vi "Main.vi"(11 "Module Admin":refnum<class "Delacor_lib_QMH_Cloneable Module Admin.lvclass">) -> ()   [LabVIEW 2020, in "Mensajes.lvlib"]
doc: "This template is based off of the Queued Message Handler design pattern and the Queued Message Handler project template that ships with LabVIEW.\n\nThe main difference is that the queue is private to this module and communication between modules is performed via Broadcast and Request events.\n\nRequest events are wrapped in public API methods and are handled in the Event Handling Loop (EHL) of this VI. Any module can register for Broadcast events sent by this module. The EHL generates messages based on user interface actions.\n\nThe Message Handling Loop (MHL) processes messages generated by the EHL, or by other messages. The messages are string values, so new messages can be added easily to the Message Cases case structure in the MHL. Each message cluster can also provide an optional value for Message Data, which is a variant that can be converted to whatever message-specific data is required.\n_____\nBased on DQMH Dev Tools: Project Template 7.1.0.1503."
uses:
  Mensajes.lvlib
  <vilib>/Delacor/Delacor QMH/Libraries/Cloneable Module Admin_class/Delacor_lib_QMH_Cloneable Module Admin.lvclass
  C:/Program Files (x86)/National Instruments/LabVIEW 2024/vi.lib/Delacor/Delacor QMH/Libraries/Module Admin_class/Delacor_lib_QMH_Module Admin.lvclass
  Module Data--cluster.ctl
  <vilib>/Delacor/Delacor QMH/Libraries/Cloneable Module Admin_class/Delacor_lib_QMH_Cloneable Module Admin.lvclass/Delacor_lib_QMH_Cloneable Module Admin.ctl
  Stop Argument--cluster.ctl
  <vilib>/Delacor/Delacor QMH/Libraries/Message Queue_class/Delacor_lib_QMH_Message Queue.lvclass/Delacor_lib_QMH_Message Queue.ctl
  <vilib>/Delacor/Delacor QMH/Libraries/Module Admin_class/Delacor_lib_QMH_Module Admin.lvclass/Delacor_lib_QMH_Module Admin.ctl
  Draw FP in Subpanel Argument--cluster.ctl
  Remove From Subpanel Argument--cluster.ctl
  Set Font Settings Argument--cluster.ctl
  <vilib>/Utility/miscctls.llb/LVFontTypeDef.ctl
  Set Message Argument--cluster.ctl
  Append String Argument--cluster.ctl
  DisplayStyle--enum.ctl
  Set Display Style Argument--cluster.ctl
  <vilib>/Utility/miscctls.llb/LVPointTypeDef.ctl
  <vilib>/Delacor/Delacor QMH/Libraries/Cloneable Module Admin_class/Delacor_lib_QMH_Get Module ID.vi
  <vilib>/Delacor/Delacor QMH/Libraries/Message Queue_class/Delacor_lib_QMH_Enqueue Message (Single).vi
  <vilib>/Delacor/Delacor QMH/Libraries/Module Admin_class/Delacor_lib_QMH_Get External Launch.vi
  <vilib>/Delacor/Delacor QMH/Libraries/Message Queue_class/Delacor_lib_QMH_Message Queue.lvclass
panel:
  out "Message":string
  out "error out":errorcluster
  out "Status":string
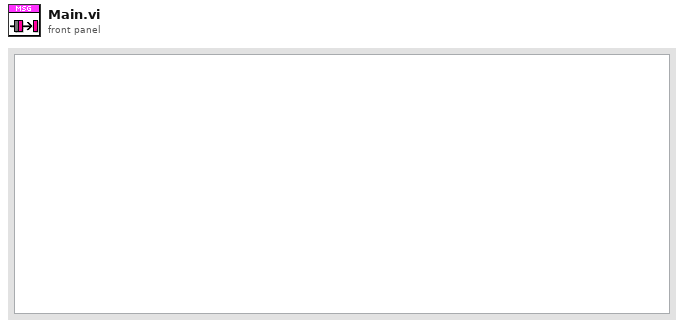
[diagram p1: front panel]
types:
  T1 = typedef "Mensajes.lvlib/Request Events--cluster.ctl" = cluster{"Stop Module":refnum<user-event>, "Show Panel":refnum<user-event>, "Hide Panel":refnum<user-event>, "Show Diagram":refnum<user-event>, "Get Module Execution Status":refnum<user-event>, "Draw FP in Subpanel":refnum<user-event>, "Remove From Subpanel":refnum<user-event>, "Set Font Settings":refnum<user-event>, "Set Message":refnum<user-event>, "Append String":refnum<user-event>, "Set Display Style":refnum<user-event>}
  T2 = typedef "Mensajes.lvlib/Module Data--cluster.ctl" = cluster{"Status":string, "Sub Panel":refnum<vi>, "Message Ref":refnum<vi>}
  T3 = enum32{"invalid lock state", "Not Locked", "Locked (No Password)", "Password-protected"}
  T4 = typedef "Mensajes.lvlib/Stop Argument--cluster.ctl" = cluster{"Module ID":i32, "Origin":string, "Exit via Stop Module Req?":bool, "Wait for Module to stop?":bool}
  T5 = typedef "Mensajes.lvlib/Draw FP in Subpanel Argument--cluster.ctl" = cluster{"Module ID":i32, "Sub Panel":refnum<vi>}
  T6 = typedef "Mensajes.lvlib/Remove From Subpanel Argument--cluster.ctl" = cluster{"Module ID":i32, "Boolean":bool}
  T7 = typedef "Mensajes.lvlib/Set Font Settings Argument--cluster.ctl" = cluster{"Module ID":i32, "Text.Font":T8}
  T8 = typedef "LVFontTypeDef.ctl" = cluster{"Font Name":string, "Size":u16, "Bold":bool, "Italic":bool, "Underline":bool, "Strikeout":bool, "Color":u32}
  T9 = typedef "Mensajes.lvlib/Set Message Argument--cluster.ctl" = cluster{"Module ID":i32, "Message":string}
  T10 = typedef "Mensajes.lvlib/Append String Argument--cluster.ctl" = cluster{"Module ID":i32, "String to Append":string}
  T11 = typedef "Mensajes.lvlib/DisplayStyle--enum.ctl" = enum16{"Normal", "Backslash", "Password", "Hexadecimal"}
  T12 = typedef "Mensajes.lvlib/Set Display Style Argument--cluster.ctl" = cluster{"Module ID":i32, "Display Style":T11}
  T13 = typedef "LVPointTypeDef.ctl" = cluster{"Horizontal":i16, "Vertical":i16}
  T14 = enum32{"Invalid", "Standard", "Closed", "Hidden", "Minimized", "Maximized"}
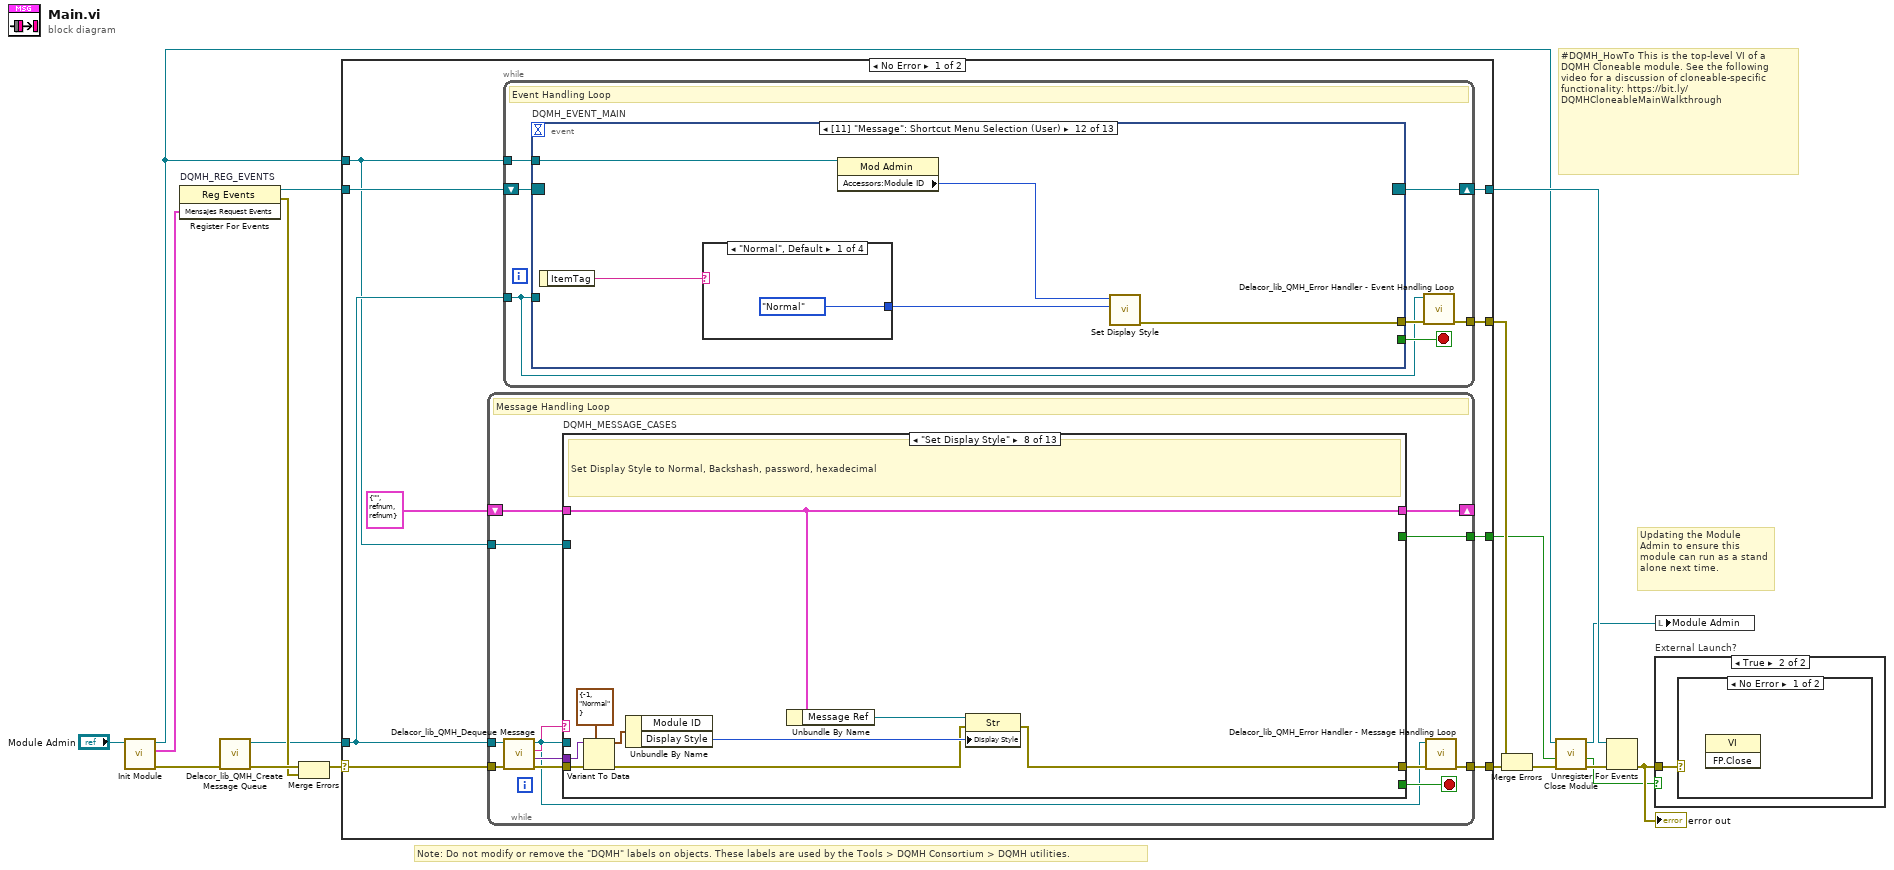
[diagram p0: block diagram]
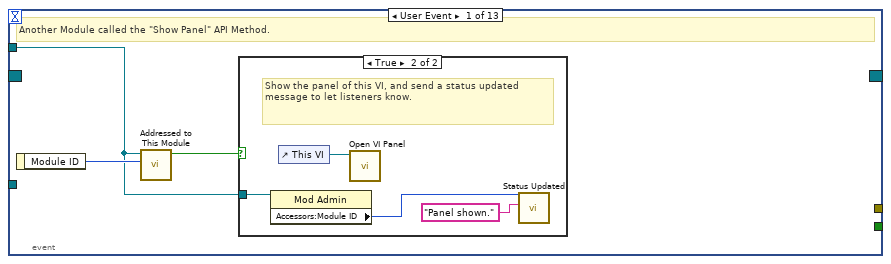
[diagram p2: hidden frame]
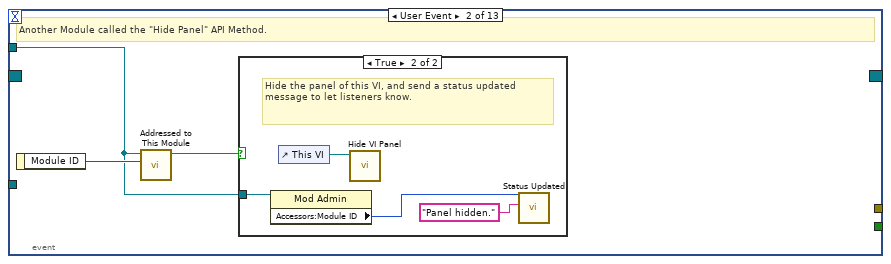
[diagram p4: hidden frame]
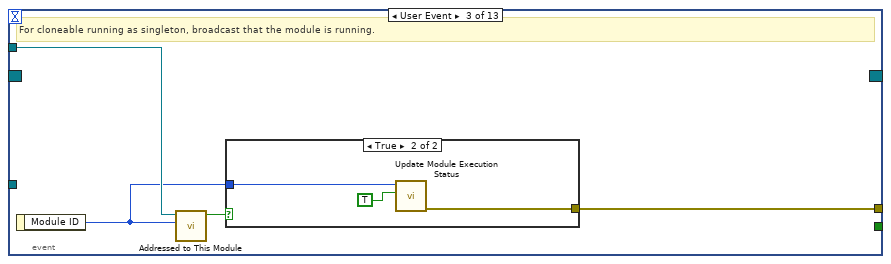
[diagram p6: hidden frame]
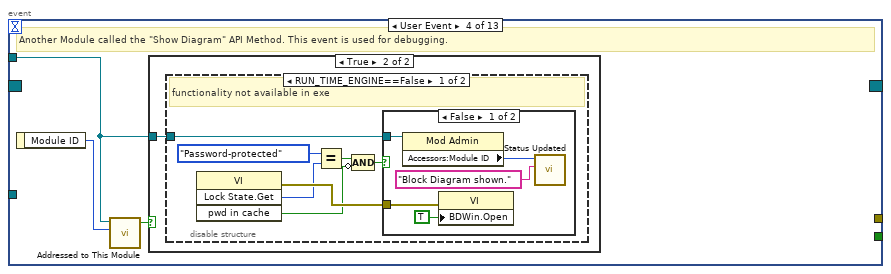
[diagram p8: hidden frame]
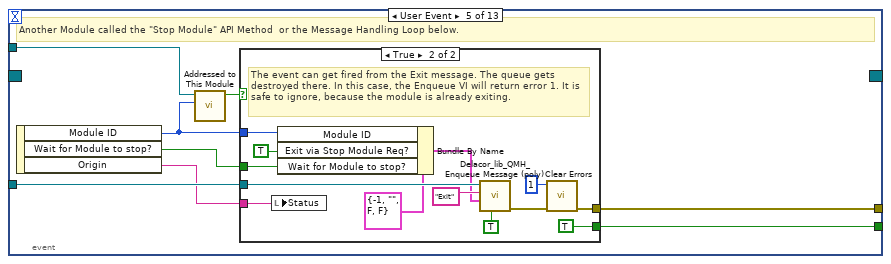
[diagram p12: hidden frame]
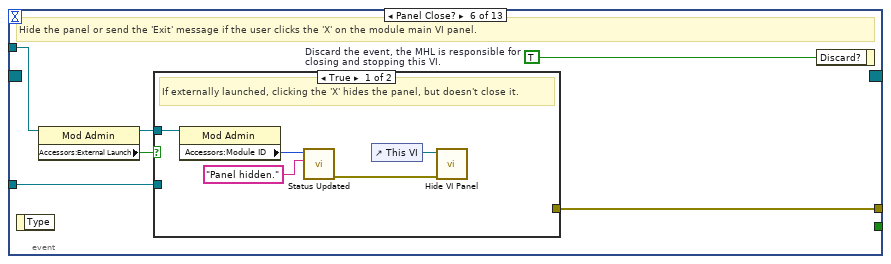
[diagram p14: hidden frame]
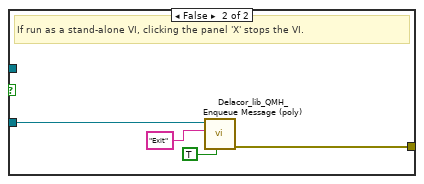
[diagram p15: hidden frame]
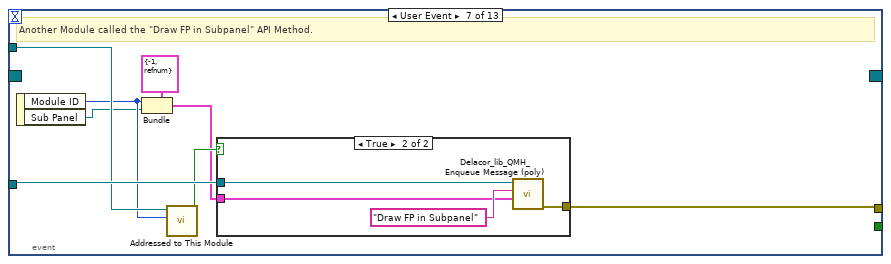
[diagram p16: hidden frame]
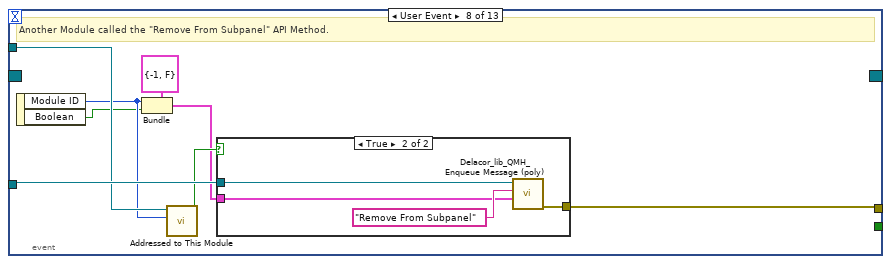
[diagram p18: hidden frame]
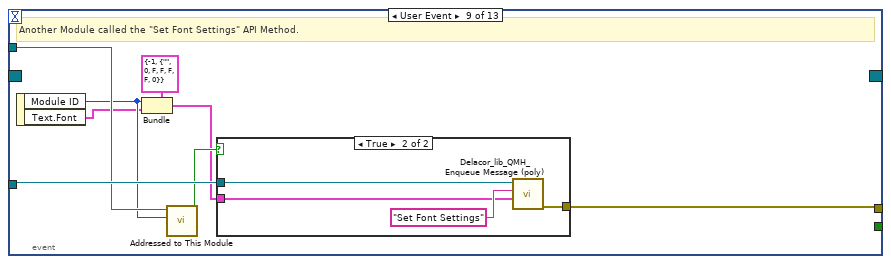
[diagram p20: hidden frame]
diagram:
  # "#DQMH_HowTo This is the top-level VI of a DQMH Cloneable module. See the following video for a discussion of cloneable-specific functionality: https://bit.ly/DQMHCloneableMainWalkthrough"
  # "Note: Do not modify or remove the \"DQMH\" labels on objects. These labels are used by the Tools > DQMH Consortium > DQMH utilities."
  # "Updating the Module Admin to ensure this module can run as a stand alone next time."
  n1 = call "Init Module.vi"("Cloneable Module Admin in"="Module Admin") -> ("error out"=w15:errorcluster, "Mensajes Request Events"=w7:T1, "Cloneable Module Admin out"=w4:refnum<class "Delacor_lib_QMH_Cloneable Module Admin.lvclass">)  [unwired: 8 in]
  n2 = register-events "DQMH_REG_EVENTS"(w7) -> (reference out=w8:refnum<event-registration>, error out=w10:errorcluster)  [unwired: 2 in]
  n3 = call <vilib>:"Delacor_lib_QMH_Create Message Queue.vi"("error in"=w15) -> ("error out"=w12:errorcluster, "Message Queue"=w6:refnum<class "Delacor_lib_QMH_Message Queue.lvclass">)  [unwired: 9 in]
  n4 = Merge Errors(w12, w10) -> (w11:errorcluster)
  n5 = case shown="No Error" w11 {
    selector: w11 -> [w25 w375]
    tunnel: [w27 w374] -> w16
    tunnel: [w24 w373] -> w9
    tunnel: w8 -> [w22 w373]
    tunnel: w6 -> [w21 w366]
    tunnel: [w26 _] -> w17
    tunnel: w4 -> [w20 w369]
    tunnel: [w19 _] -> w2
    frame No Error {
      n6 = while {
        tunnel: w21 -> [w189]
        shift-right: [w196] -> _
        shift-left: T2 {"Status"="", "Sub Panel"=refnum, "Message Ref"=refnum} ("Data Cluster") -> [w197]
        tunnel: w25 -> [w200]
        tunnel: [w198] -> w27
        tunnel: w20 -> [w191]
        tunnel: [w190] -> w19
        stop <- w195 stop-if-true
        # "Message Handling Loop"
        n7 = call-dynamic "Delacor_lib_QMH_Dequeue Message.vi"("error in"=w200, "Message Queue in"=w189) -> ("error out"=w199:errorcluster, "Message Data"=w193:variant, "Message"=w194:string, "Message Queue out"=w192:refnum<class "Delacor_lib_QMH_Message Queue.lvclass">)  [unwired: 6 in]
        n8 = case "DQMH_MESSAGE_CASES" shown="\"Set Display Style\"" w194 {
          selector: w194 -> [_ _ _ _ _ _ _ _ _ _ _ _ w355]
          tunnel: w192 -> [_ _ _ _ _ _ _ _ _ _ w319 w347 _]
          tunnel: w199 -> [w221 w225 w244 w264 w279 w290 w303 w312 w315 w317 w329 w353 w364]
          tunnel: [w219 w225 w240 w262 w274 w288 w298 w306 w314 w317 w325 w348 w365] -> w201
          tunnel: w197 -> [w212 w224 w230 w256 w272 w289 w297 w305 w313 w316 w323 w337 w362]
          tunnel: [w211 w224 w231 w252 w272 w289 w297 w305 w313 w316 w323 w337 w362] -> w196
          tunnel: [_ _ _ _ _ _ _ _ _ _ _ w346 _] -> w195
          tunnel: w193 -> [_ _ w239 w261 w278 w287 w302 w311 _ _ w322 w344 _]
          tunnel: w191 -> [w207 _ w228 w255 _ w284 w294 _ _ _ w321 w339 w361]
          tunnel: [_ _ _ _ _ _ _ _ _ _ _ w342 _] -> w190
          frame "Initialize" {
            w204 = "Initial Message" ("Initial Message")
            # "Initialize - Any operation that needs to be done before the module can receive messages. Synchronize Caller Events.vi will inform Start Module.vi that the module has launched and is ready to receive messages. Module Did Init.vi will broadcast that the module initialized."
            n9 = call "Synchronize Caller Events.vi"("error in"=w221, "Module Admin"=w207) -> ("error out"=w220:errorcluster, "Module Admin out"=w206:refnum<class "Delacor_lib_QMH_Cloneable Module Admin.lvclass">)  [unwired: 8 in]
            n10 = property on="Property Node" class="Mod Admin"(reference=w206) -> ("Accessors:Module ID"=w203:i32, "Accessors:External Launch"=w208:bool)  [unwired: 1 in, 2 out]
            n11 = call "Module Name--constant.vi"("Module ID"=w203) -> ("Module Name"=w216:string)  [unwired: 10 in]
            n12 = property on="Property Node" class="VI"("Front Panel.Title"=w216) -> (reference out=w218:refnum<vi>, error out=w223:errorcluster)  [unwired: 2 in]
            n13 = Select(t=T14."Hidden" ("State"), s=w208, f=T14."Standard" ("State")) -> (s? t:f=w213:T14)
            n14 = control-ref of="Message"() -> (w202:refnum<vi>)
            n15 = invoke on="Invoke Node" class="VI" method="FP.Open"(reference=w218, error in=w223, "State"=w213) -> (reference out=w217:refnum<vi>, error out=w222:errorcluster)  [unwired: 2 in, 3 out]
            n16 = Bundle By Name(cluster=w212, "Message Ref"=w202, "Status"=w204) -> (w211:T2)
            n17 = invoke on="Invoke Node" class="VI" method="FP.Center"(reference=w217, error in=w222) -> ()  [unwired: 1 in, 3 out]
            n18 = property on="Pane" class="Pane"("Origin"=T13 {"Horizontal"=0, "Vertical"=0}) -> ()  [unwired: 2 in, 2 out]
            n19 = call "Module Name--constant.vi"("Module ID"=w203) -> ("Module Name"=w209:string)  [unwired: 10 in]
            n20 = call "Module Did Init.vi"("error in"=w220, "Initialized?"=TRUE, "Origin"=w209, "Module ID"=w203) -> ("error out"=w219:errorcluster)  [unwired: 7 in]
            "Status" <- w204
          }
          frame "---Module Specific---" {
            # "Separator -- The following cases handle messages specific to this Module."
          }
          frame "Draw FP in Subpanel" {
            # "Draw FP in Subpanel"
            n21 = Variant To Data(error in=w244, type=T5 {"Module ID"=-1, "Sub Panel"=refnum} ("Draw FP in Subpanel Argument"), Variant=w239) -> (data=w237:T5, error out=w241:errorcluster)
            n22 = property class="Mod Admin"(reference=w228) -> ("Accessors:Module ID"=w227:i32)  [unwired: 1 in, 2 out]
            n23 = Unbundle By Name(w237) -> ("Sub Panel"=w229:refnum<vi>)
            n24 = control-ref of="This VI"() -> (w234:refnum<vi>)
            n25 = property class="VI"(reference=w234, error in=w241) -> (reference out=w233:refnum<vi>, error out=w242:errorcluster, "FP.State"=w232:T14)
            n26 = case shown="\"Closed\"" w232 {
              tunnel: [w245 w248] -> w235
              tunnel: [w246 w250] -> w243
              tunnel: w242 -> [w246 w249]
              tunnel: w233 -> [w245 w247]
              frame "Closed" {
              }
              frame "Standard", Default {
                n27 = invoke class="VI" method="FP.Close"(reference=w247, error in=w249) -> (reference out=w248:refnum<vi>, error out=w250:errorcluster)  [unwired: 1 in, 1 out]
              }
            }
            n28 = invoke class="SubPnl" method="Insert VI"(reference=w229, error in=w243, "VI Ref"=w235) -> (reference out=w236:refnum<vi>, error out=w240:errorcluster)  [unwired: 1 in, 2 out]
            n29 = call "Status Updated.vi"("error in"=w240, "Status"="Front Panel Inserted in Subpanel", "Module ID"=w227) -> ()  [unwired: 8 in, 1 out]
            n30 = Bundle By Name(cluster=w230, "Sub Panel"=w236) -> (w231:T2)
          }
          frame "Remove From Subpanel" {
            # "Remove From Subpanel"
            n31 = Variant To Data(error in=w264, type=T6 {"Module ID"=-1, "Boolean"=FALSE} ("Remove From Subpanel Argument"), Variant=w261) -> (data=w259:T6, error out=w263:errorcluster)
            n32 = Unbundle By Name(w259) -> ()  [unwired: 2 out]
            n33 = property class="Mod Admin"(reference=w255) -> ("Accessors:Module ID"=w254:i32)  [unwired: 1 in, 2 out]
            n34 = Unbundle By Name(w256) -> ("Sub Panel"=w258:refnum<vi>)
            n35 = Not A Number/Path/Refnum?(number/path/refnum=w258) -> (NaN/Path/Refnum?=w257:bool)
            n36 = case shown="False" w257 {
              tunnel: w263 -> [w268 w270]
              tunnel: [w267 w270] -> w262
              tunnel: w258 -> [w266 _]
              tunnel: ["Panel Removed from Subpanel" "This module has not been inserted into the subpanel"] -> w253
              frame False {
                n37 = invoke class="SubPnl" method="Remove VI"(reference=w266, error in=w268) -> (error out=w267:errorcluster)  [unwired: 1 in, 2 out]
              }
              frame True {
              }
            }
            n38 = Bundle By Name(cluster=w256, "Sub Panel"=refnum<vi> refnum) -> (w252:T2)
            n39 = call "Status Updated.vi"("error in"=w262, "Status"=w253, "Module ID"=w254) -> ()  [unwired: 8 in, 1 out]
          }
          frame "Set Font Settings" {
            # "Set Font Name, Size, Bold, Italic, Underline, Strikeout, and Color"
            n40 = Variant To Data(error in=w279, type=T7 {"Module ID"=-1, "Text.Font"={"Font Name"="", "Size"=0, "Bold"=FALSE, "Italic"=FALSE, "Underline"=FALSE, "Strikeout"=FALSE, "Color"=0}} ("Set Font Settings Argument"), Variant=w278) -> (data=w276:T7, error out=w275:errorcluster)
            n41 = Unbundle By Name(w276) -> ("Text.Font"=w273:T8)  [unwired: 1 out]
            n42 = Unbundle By Name(w272) -> ("Message Ref"=w271:refnum<vi>)
            n43 = property class="Str"(reference=w271, error in=w275, "Text.Font"=w273) -> (error out=w274:errorcluster)  [unwired: 1 out]
          }
          frame "Set Message" {
            # "Set Message"
            n44 = Variant To Data(error in=w290, type=T9 {"Module ID"=-1, "Message"=""} ("Set Message Argument"), Variant=w287) -> (data=w285:T9, error out=w288:errorcluster)
            n45 = property class="Mod Admin"(reference=w284) -> ("Accessors:Module ID"=w283:i32)  [unwired: 1 in, 2 out]
            n46 = Unbundle By Name(w285) -> ("Message"=w282:string)
            "Message" <- w282
            n47 = Format Into String(format string="Message Set: %s", w282) -> (resulting string=w281:string)  [unwired: 2 in, 1 out]
            n48 = call "Status Updated.vi"("Status"=w281, "Module ID"=w283) -> ()  [unwired: 9 in, 1 out]
          }
          frame "Append String" {
            # "Append String"
            n49 = Variant To Data(error in=w303, type=T10 {"Module ID"=-1, "String to Append"=""} ("Append String Argument"), Variant=w302) -> (data=w300:T10, error out=w299:errorcluster)
            n50 = Unbundle By Name(w300) -> ("String to Append"=w293:string)  [unwired: 1 out]
            n51 = property class="Mod Admin"(reference=w294) -> ("Accessors:Module ID"=w295:i32)  [unwired: 1 in, 2 out]
            n52 = Unbundle By Name(w297) -> ("Message Ref"=w296:refnum<vi>)
            n53 = Format Into String(format string="Appending String: %s", w293) -> (resulting string=w292:string)  [unwired: 2 in, 1 out]
            n54 = invoke class="Str" method="Append String"(reference=w296, error in=w299, "string"=w293) -> (error out=w298:errorcluster)  [unwired: 1 in, 3 out]
            n55 = call "Status Updated.vi"("Status"=w292, "Module ID"=w295) -> ()  [unwired: 9 in, 1 out]
          }
          frame "Set Display Style" {
            # "Set Display Style to Normal, Backshash, password, hexadecimal"
            n56 = Variant To Data(error in=w312, type=T12 {"Module ID"=-1, "Display Style"=enum."Normal"} ("Set Display Style Argument"), Variant=w311) -> (data=w309:T12, error out=w307:errorcluster)
            n57 = Unbundle By Name(w309) -> ("Display Style"=w308:T11)  [unwired: 1 out]
            n58 = Unbundle By Name(w305) -> ("Message Ref"=w304:refnum<vi>)
            n59 = property class="Str"(reference=w304, error in=w307, "Display Style"=w308) -> (error out=w306:errorcluster)  [unwired: 1 out]
          }
          frame "---Copy This Frame---" {
            # "Duplicate this frame when creating new messages.  Change this comment in the duplicated frame to describe this message."
            n60 = Merge Errors(w315) -> (w314:errorcluster)
          }
          frame "---Exit and Error Handling---" {
            # "Separator - the following cases handle errors and exit messages."
          }
          frame "Error" {
            # "#DQMH_CodeRecommended - If the module is running in standalone mode (External Launch = FALSE), this code will pop up an error dialog and call the 'Exit' message if an error occurs. Add more fine-grained error management here."
            # "Error - Check the error message data and respond accordingly. This message is sent by the \"Error Handler\" VIs at the end of each loop in this application."
            n61 = property on="Property Node" class="Mod Admin"(reference=w321) -> ("Accessors:External Launch"=w320:bool, "Accessors:Module ID"=w318:i32)  [unwired: 1 in, 2 out]
            n62 = Variant To Data(error in=w329, type=errorcluster {"status"=FALSE, "code"=0, "source"=""} ("error constant"), Variant=w322) -> (data=w324:errorcluster, error out=w327:errorcluster)
            n63 = local write "error out"(w324) -> ()
            n64 = call "Error Reported.vi"("Error"=w324, "Module ID"=w318) -> ()  [unwired: 9 in, 1 out]
            n65 = case shown="False" w320 {
              tunnel: [w334 _] -> w326
              tunnel: w319 -> [w332 _]
              tunnel: w324 -> [w333 _]
              frame False {
                n66 = disable-structure shown="Default" {
                  disable-tunnel: w333 -> [w335 _]
                  frame condition #0 (active) {
                    # "If the module is running standalone, then pop up an error dialog and call the \"Exit\" message."
                    n67 = call <vilib>:"Simple Error Handler.vi"("error in (no error)"=w335) -> ()  [unwired: 4 in, 5 out]
                  }
                  frame condition #1 {
                    # "To prevent the Simple Error Handler VI from being loaded (e.g. when deploying to a Real-Time target), add the Conditional Disable Symbol \"DQMH_Disable_SEH\" to your project and set it to TRUE."
                  }
                }
                n68 = call-poly <vilib>:"Delacor_lib_QMH_Enqueue Message (poly).vi"("Priority Message? (F)"=TRUE, "Message"="Exit", "Message Queue in"=w332) -> ("error out"=w334:errorcluster)  [unwired: 7 in, 1 out]
              }
              frame True {
                # "If the module was launched externally, calling the Error Reported broadcast VI is the only action performed by the \"Error\" message. The module's caller can then process the error appropriately."
              }
            }
            n69 = Merge Errors(w327, w326) -> (w325:errorcluster)
          }
          frame "Exit" {
            w345 = 91  # 91: not all Exit messages will have an argument
            w346 = TRUE  # Stop the VI
            # "Release the message queue reference"
            # "#DQMH_CodeNeeded - Add any required cleanup code here."
            # "Exit - Exit the application."
            n70 = Variant To Data(error in=w353, type=T4 {"Module ID"=-1, "Origin"="", "Exit via Stop Module Req?"=FALSE, "Wait for Module to stop?"=FALSE} ("Stop Argument"), Variant=w344) -> (data=w341:T4, error out=w349:errorcluster)
            n71 = call <vilib>:"Clear Errors.vi"("error in (no error)"=w349, "specific error code to clear (0: all)"=w345) -> ("error out"=w352:errorcluster)  [unwired: 4 in, 1 out]
            n72 = property on="Property Node" class="Mod Admin"(reference=w339) -> ("Accessors:Module ID"=w338:i32)  [unwired: 1 in, 2 out]
            n73 = control-ref of="This VI"() -> (w340:refnum<vi>)
            n74 = call-dynamic "Delacor_lib_QMH_Release Message Queue.vi"("error in"=w352, "Message Queue"=w347) -> ("error out"=w351:errorcluster)  [unwired: 9 in]
            n75 = call "Handle Exit.vi"("Stop Argument"=w341, "Module Admin in"=w339, "VI reference"=w340) -> ("error out"=w350:errorcluster, "Wait for Stop?"=w342:bool)  [unwired: 7 in]
            n76 = Merge Errors(w351, w350) -> (w348:errorcluster)
            n77 = Unbundle By Name(w337) -> ("Sub Panel"=w336:refnum<vi>)
            n78 = call "Error Reported.vi"("Error"=w348, "Module ID"=w338) -> ()  [unwired: 9 in, 1 out]
            n79 = invoke class="SubPnl" method="Remove VI"(reference=w336) -> ()  [unwired: 2 in, 3 out]
          }
          frame Default {
            # "'Default' case only runs if there is a message that isn't defined in any of the other cases.  Output a programming error."
            n80 = property on="Property Node" class="Mod Admin"(reference=w361) -> ("Accessors:Module ID"=w360:i32)  [unwired: 1 in, 2 out]
            n81 = call "Module Name--constant.vi"("Module ID"=w360) -> ("Module Name"=w354:string)  [unwired: 10 in]
            n82 = Format Into String(format string="The invalid message string \"%s\" was received in the Message Handling Loop for module \"%s\".", w355, w354) -> (resulting string=w357:string)  [unwired: 2 in, 1 out]
            n83 = call <vilib>:"Error Cluster From Error Code.vi"("show call chain? (False)"=TRUE, "error message (\"\")"=w357, "error code (0)"=1) -> ("error out"=w363:errorcluster)  [unwired: 6 in]
            n84 = Merge Errors(w364, w363) -> (w365:errorcluster)
          }
        }
        n85 = call-dynamic "Delacor_lib_QMH_Error Handler - Message Handling Loop.vi"("error in"=w201, "Message Queue in"=w192) -> ("dup error in"=w198:errorcluster)  [unwired: 8 in, 1 out]
      }
      n86 = while {
        tunnel: w21 -> [w28]
        shift-right: [w31] -> w24
        shift-left: w22 -> [w32]
        tunnel: [w33] -> w26
        tunnel: w20 -> [w29]
        stop <- w30 stop-if-true
        # "Event Handling Loop"
        n87 = event "DQMH_EVENT_MAIN" shown="[11] \"Message\": Shortcut Menu Selection (User)" {
          selector: w32 -> [_ _ _ _ _ _ _ _ _ _ _ _ _]
          dyn-events: [_ _ _ _ _ _ _ _ _ _ _ _ _] -> w31
          timeout: _ -> [_ _ _ _ _ _ _ _ _ _ _ _ _]
          tunnel: [_ _ _ _ w75 _ _ _ _ _ _ _ _] -> w30
          tunnel: w28 -> [_ _ _ _ w78 w95 w114 w126 w139 w151 w163 _ w184]
          tunnel: [_ _ w52 _ w79 w98 w115 w127 w132 w144 w156 w168 w177] -> w34
          tunnel: w29 -> [w35 w42 w50 w56 w77 w96 w112 w124 w137 w149 w161 w172 w182]
          event User Event {
            # "Another Module called the \"Show Panel\" API Method."
            n88 = event-data() -> ("Module ID"=w36:i32)  [unwired: 1 in]
            n89 = call "Addressed to This Module.vi"("Module ID from Argument"=w36, "Module Admin"=w35) -> ("Addressed to this instance?"=w37:bool)  [unwired: 8 in, 1 out]
            n90 = case shown="True" w37 {
              tunnel: w35 -> [_ w39]
              frame False {
              }
              frame True {
                # "Show the panel of this VI, and send a status updated message to let listeners know."
                n91 = property on="Property Node" class="Mod Admin"(reference=w39) -> ("Accessors:Module ID"=w38:i32)  [unwired: 1 in, 2 out]
                n92 = control-ref of="This VI"() -> (w41:refnum<vi>)
                n93 = call "Open VI Panel.vi"("VI"=w41) -> ()  [unwired: 10 in, 1 out]
                n94 = call "Status Updated.vi"("Status"="Panel shown." ("format string"), "Module ID"=w38) -> ()  [unwired: 9 in, 1 out]
              }
            }
          }
          event User Event {
            # "Another Module called the \"Hide Panel\" API Method."
            n95 = event-data() -> ("Module ID"=w43:i32)  [unwired: 1 in]
            n96 = call "Addressed to This Module.vi"("Module ID from Argument"=w43, "Module Admin"=w42) -> ("Addressed to this instance?"=w44:bool)  [unwired: 8 in, 1 out]
            n97 = case shown="True" w44 {
              tunnel: w42 -> [_ w46]
              frame False {
              }
              frame True {
                # "Hide the panel of this VI, and send a status updated message to let listeners know."
                n98 = property on="Property Node" class="Mod Admin"(reference=w46) -> ("Accessors:Module ID"=w45:i32)  [unwired: 1 in, 2 out]
                n99 = control-ref of="This VI"() -> (w48:refnum<vi>)
                n100 = call "Hide VI Panel.vi"("VI"=w48) -> ()  [unwired: 10 in, 1 out]
                n101 = call "Status Updated.vi"("Status"="Panel hidden." ("format string"), "Module ID"=w45) -> ()  [unwired: 9 in, 1 out]
              }
            }
          }
          event User Event {
            # "For cloneable running as singleton, broadcast that the module is running."
            n102 = event-data() -> ("Module ID"=w49:i32)  [unwired: 1 in]
            n103 = call "Addressed to This Module.vi"("Module ID from Argument"=w49, "Module Admin"=w50) -> ("Addressed to this instance?"=w51:bool)  [unwired: 8 in, 1 out]
            n104 = case shown="True" w51 {
              tunnel: [_ w55] -> w52
              tunnel: w49 -> [_ w54]
              frame False {
              }
              frame True {
                n105 = call "Update Module Execution Status.vi"("Running?"=TRUE, "Module ID"=w54) -> ("error out"=w55:errorcluster)  [unwired: 9 in]
              }
            }
          }
          event User Event {
            # "Another Module called the \"Show Diagram\" API Method. This event is used for debugging."
            n106 = event-data() -> ("Module ID"=w57:i32)  [unwired: 1 in]
            n107 = call "Addressed to This Module.vi"("Module ID from Argument"=w57, "Module Admin"=w56) -> ("Addressed to this instance?"=w58:bool)  [unwired: 8 in, 1 out]
            n108 = case shown="True" w58 {
              tunnel: w56 -> [_ w59]
              frame False {
              }
              frame True {
                n109 = disable-structure shown="RUN_TIME_ENGINE==False" {
                  disable-tunnel: w59 -> [w60 _]
                  frame condition #0 (active) {
                    # "functionality not available in exe"
                    n110 = invoke on="Invoke Node" class="VI" method="Lock State.Get"() -> (error out=w66:errorcluster, "Get Lock State"=w65:T3, "pwd in cache"=w62:bool)  [unwired: 4 in, 1 out]
                    n111 = Equal?(x=T3."Password-protected", y=w65) -> (x = y?=w63:bool)
                    n112 = Compound Arithmetic op=AND(w63, invert w62) -> (w61:bool)
                    n113 = case shown="False" w61 {
                      tunnel: w66 -> [w71 _]
                      tunnel: w60 -> [w68 _]
                      frame False {
                        n114 = property on="Property Node" class="Mod Admin"(reference=w68) -> ("Accessors:Module ID"=w67:i32)  [unwired: 1 in, 2 out]
                        n115 = property on="Property Node" class="VI"(error in=w71, "BDWin.Open"=TRUE ("Block Diagram Window:Open")) -> ()  [unwired: 1 in, 2 out]
                        n116 = call "Status Updated.vi"("Status"="Block Diagram shown." ("format string"), "Module ID"=w67) -> ()  [unwired: 9 in, 1 out]
                      }
                      frame True {
                        # "Password-protected VI, and the password is not in the cache. Do not show the diagram."
                      }
                    }
                  }
                  frame condition #1 {
                  }
                }
              }
            }
          }
          event User Event {
            # "Another Module called the \"Stop Module\" API Method  or the Message Handling Loop below."
            n117 = event-data() -> ("Module ID"=w73:i32, "Wait for Module to stop?"=w74:bool, "Origin"=w72:string)  [unwired: 1 in]
            n118 = call "Addressed to This Module.vi"("Module ID from Argument"=w73, "Module Admin"=w77) -> ("Addressed to this instance?"=w76:bool)  [unwired: 8 in, 1 out]
            n119 = case shown="True" w76 {
              tunnel: [_ w91] -> w79
              tunnel: w78 -> [_ w87]
              tunnel: [_ TRUE] -> w75
              tunnel: w74 -> [_ w82]
              tunnel: w73 -> [_ w84]
              tunnel: w72 -> [_ w80]
              frame False {
              }
              frame True {
                # "The event can get fired from the Exit message. The queue gets destroyed there. In this case, the Enqueue VI will return error 1. It is safe to ignore, because the module is already exiting."
                n120 = local write "Status"(w80) -> ()
                n121 = Bundle By Name(cluster=T4 {"Module ID"=-1, "Origin"="", "Exit via Stop Module Req?"=FALSE, "Wait for Module to stop?"=FALSE} ("Stop Argument"), "Module ID"=w84, "Exit via Stop Module Req?"=TRUE, "Wait for Module to stop?"=w82) -> (w81:T4)
                n122 = call-poly <vilib>:"Delacor_lib_QMH_Enqueue Message (poly).vi"("Priority Message? (F)"=TRUE, "Message Data"=w81, "Message"="Exit", "Message Queue in"=w87) -> ("error out"=w92:errorcluster)  [unwired: 6 in, 1 out]
                n123 = call <vilib>:"Clear Errors.vi"("error in (no error)"=w92, "specific error code to clear (0: all)"=1) -> ("error out"=w91:errorcluster)  [unwired: 4 in, 1 out]
              }
            }
          }
          event Panel Close? {
            w97 = TRUE  # Discard the event, the MHL is responsible for closing and stopping this VI.
            # "Hide the panel or send the 'Exit' message if the user clicks the 'X' on the module main VI panel."
            n124 = event-data() -> ()  [unwired: 1 in, 1 out]
            n125 = property on="Property Node" class="Mod Admin"(reference=w96) -> (reference out=w93:refnum<class "Delacor_lib_QMH_Cloneable Module Admin.lvclass">, "Accessors:External Launch"=w94:bool)  [unwired: 1 in, 1 out]
            n126 = case shown="True" w94 {
              tunnel: w95 -> [_ w106]
              tunnel: [_ w107] -> w98
              tunnel: w93 -> [w100 _]
              frame True {
                # "If externally launched, clicking the 'X' hides the panel, but doesn't close it."
                n127 = property on="Property Node" class="Mod Admin"(reference=w100) -> ("Accessors:Module ID"=w99:i32)  [unwired: 1 in, 2 out]
                n128 = call "Status Updated.vi"("Status"="Panel hidden." ("format string"), "Module ID"=w99) -> ("error out"=w103:errorcluster)  [unwired: 9 in]
                n129 = control-ref of="This VI"() -> (w102:refnum<vi>)
                n130 = call "Hide VI Panel.vi"("error in"=w103, "VI"=w102) -> ()  [unwired: 9 in, 1 out]
              }
              frame False {
                # "If run as a stand-alone VI, clicking the panel 'X' stops the VI."
                n131 = call-poly <vilib>:"Delacor_lib_QMH_Enqueue Message (poly).vi"("Priority Message? (F)"=TRUE, "Message"="Exit", "Message Queue in"=w106) -> ("error out"=w107:errorcluster)  [unwired: 7 in, 1 out]
              }
            }
            n132 = event-data ("Event Filter Node")("Discard?"=w97) -> ()  [unwired: 1 in, 1 out]
          }
          event User Event {
            # "Another Module called the \"Draw FP in Subpanel\" API Method."
            n133 = event-data() -> ("Module ID"=w109:i32, "Sub Panel"=w108:refnum<vi>)  [unwired: 1 in]
            n134 = Bundle(cluster=T5 {"Module ID"=-1, "Sub Panel"=refnum} ("Draw FP in Subpanel Argument"), "Module ID"=w109, "Sub Panel"=w108) -> (w110:T5)
            n135 = call "Addressed to This Module.vi"("Module ID from Argument"=w109, "Module Admin"=w112) -> ("Addressed to this instance?"=w113:bool)  [unwired: 8 in, 1 out]
            n136 = case shown="True" w113 {
              tunnel: w114 -> [_ w118]
              tunnel: w110 -> [_ w116]
              tunnel: [_ w119] -> w115
              frame False {
              }
              frame True {
                n137 = call-poly <vilib>:"Delacor_lib_QMH_Enqueue Message (poly).vi"("Message Data"=w116, "Message"="Draw FP in Subpanel", "Message Queue in"=w118) -> ("error out"=w119:errorcluster)  [unwired: 7 in, 1 out]
              }
            }
          }
          event User Event {
            # "Another Module called the \"Remove From Subpanel\" API Method."
            n138 = event-data() -> ("Module ID"=w121:i32, "Boolean"=w120:bool)  [unwired: 1 in]
            n139 = Bundle(cluster=T6 {"Module ID"=-1, "Boolean"=FALSE} ("Remove From Subpanel Argument"), "Module ID"=w121, "Boolean"=w120) -> (w122:T6)
            n140 = call "Addressed to This Module.vi"("Module ID from Argument"=w121, "Module Admin"=w124) -> ("Addressed to this instance?"=w125:bool)  [unwired: 8 in, 1 out]
            n141 = case shown="True" w125 {
              tunnel: w126 -> [_ w130]
              tunnel: w122 -> [_ w128]
              tunnel: [_ w131] -> w127
              frame False {
              }
              frame True {
                n142 = call-poly <vilib>:"Delacor_lib_QMH_Enqueue Message (poly).vi"("Message Data"=w128, "Message"="Remove From Subpanel", "Message Queue in"=w130) -> ("error out"=w131:errorcluster)  [unwired: 7 in, 1 out]
              }
            }
          }
          event User Event {
            # "Another Module called the \"Set Font Settings\" API Method."
            n143 = event-data() -> ("Module ID"=w134:i32, "Text.Font"=w133:T8)  [unwired: 1 in]
            n144 = Bundle(cluster=T7 {"Module ID"=-1, "Text.Font"={"Font Name"="", "Size"=0, "Bold"=FALSE, "Italic"=FALSE, "Underline"=FALSE, "Strikeout"=FALSE, "Color"=0}} ("Set Font Settings Argument"), "Module ID"=w134, "Text.Font"=w133) -> (w135:T7)
            n145 = call "Addressed to This Module.vi"("Module ID from Argument"=w134, "Module Admin"=w137) -> ("Addressed to this instance?"=w138:bool)  [unwired: 8 in, 1 out]
            n146 = case shown="True" w138 {
              tunnel: w139 -> [_ w143]
              tunnel: w135 -> [_ w141]
              tunnel: [_ w140] -> w132
              frame False {
              }
              frame True {
                n147 = call-poly <vilib>:"Delacor_lib_QMH_Enqueue Message (poly).vi"("Message Data"=w141, "Message"="Set Font Settings", "Message Queue in"=w143) -> ("error out"=w140:errorcluster)  [unwired: 7 in, 1 out]
              }
            }
          }
          event User Event {
            # "Another Module called the \"Set Message\" API Method."
            n148 = event-data() -> ("Module ID"=w146:i32, "Message"=w145:string)  [unwired: 1 in]
            n149 = Bundle(cluster=T9 {"Module ID"=-1, "Message"=""} ("Set Message Argument"), "Module ID"=w146, "Message"=w145) -> (w147:T9)
            n150 = call "Addressed to This Module.vi"("Module ID from Argument"=w146, "Module Admin"=w149) -> ("Addressed to this instance?"=w150:bool)  [unwired: 8 in, 1 out]
            n151 = case shown="True" w150 {
              tunnel: w151 -> [_ w155]
              tunnel: w147 -> [_ w153]
              tunnel: [_ w152] -> w144
              frame False {
              }
              frame True {
                n152 = call-poly <vilib>:"Delacor_lib_QMH_Enqueue Message (poly).vi"("Message Data"=w153, "Message"="Set Message", "Message Queue in"=w155) -> ("error out"=w152:errorcluster)  [unwired: 7 in, 1 out]
              }
            }
          }
          event User Event {
            # "Another Module called the \"Append String\" API Method."
            n153 = event-data() -> ("Module ID"=w158:i32, "String to Append"=w157:string)  [unwired: 1 in]
            n154 = Bundle(cluster=T10 {"Module ID"=-1, "String to Append"=""} ("Append String Argument"), "Module ID"=w158, "String to Append"=w157) -> (w159:T10)
            n155 = call "Addressed to This Module.vi"("Module ID from Argument"=w158, "Module Admin"=w161) -> ("Addressed to this instance?"=w162:bool)  [unwired: 8 in, 1 out]
            n156 = case shown="True" w162 {
              tunnel: w163 -> [_ w167]
              tunnel: w159 -> [_ w165]
              tunnel: [_ w164] -> w156
              frame False {
              }
              frame True {
                n157 = call-poly <vilib>:"Delacor_lib_QMH_Enqueue Message (poly).vi"("Message Data"=w165, "Message"="Append String", "Message Queue in"=w167) -> ("error out"=w164:errorcluster)  [unwired: 7 in, 1 out]
              }
            }
          }
          event "Message": Shortcut Menu Selection (User) {
            n158 = event-data() -> ("ItemTag"=w169:string)  [unwired: 1 in]
            n159 = case shown="\"Normal\", Default" w169 {
              tunnel: [DisplayStyle--enum."Normal" ("Display Style") DisplayStyle--enum."Backslash" ("Display Style") DisplayStyle--enum."Password" ("Display Style") DisplayStyle--enum."Hexadecimal" ("Display Style")] -> w170
              frame "Normal", Default {
              }
              frame "Backslash" {
              }
              frame "Password" {
              }
              frame "Hexadecimal" {
              }
            }
            n160 = property class="Mod Admin"(reference=w172) -> ("Accessors:Module ID"=w171:i32)  [unwired: 1 in, 2 out]
            n161 = call "Set Display Style.vi"("Display Style"=w170, "Module ID"=w171) -> ("error out"=w168:errorcluster)  [unwired: 9 in]
          }
          event User Event {
            # "Another Module called the \"Set Display Style\" API Method."
            n162 = event-data() -> ("Module ID"=w179:i32, "Display Style"=w178:T11)  [unwired: 1 in]
            n163 = Bundle(cluster=T12 {"Module ID"=-1, "Display Style"=enum."Normal"} ("Set Display Style Argument"), "Module ID"=w179, "Display Style"=w178) -> (w180:T12)
            n164 = call "Addressed to This Module.vi"("Module ID from Argument"=w179, "Module Admin"=w182) -> ("Addressed to this instance?"=w183:bool)  [unwired: 8 in, 1 out]
            n165 = case shown="True" w183 {
              tunnel: w184 -> [_ w188]
              tunnel: w180 -> [_ w186]
              tunnel: [_ w185] -> w177
              frame False {
              }
              frame True {
                n166 = call-poly <vilib>:"Delacor_lib_QMH_Enqueue Message (poly).vi"("Message Data"=w186, "Message"="Set Display Style", "Message Queue in"=w188) -> ("error out"=w185:errorcluster)  [unwired: 7 in, 1 out]
              }
            }
          }
        }
        n167 = call-dynamic "Delacor_lib_QMH_Error Handler - Event Handling Loop.vi"("error in"=w34, "Message Queue in"=w28) -> ("dup error in"=w33:errorcluster)  [unwired: 8 in, 1 out]
      }
    }
    frame Error {
      n168 = call "Synchronize Caller Events.vi"("Module Admin"=w369) -> ("Module Admin out"=w368:refnum<class "Delacor_lib_QMH_Cloneable Module Admin.lvclass">)  [unwired: 9 in, 1 out]
      n169 = property on="Property Node" class="Mod Admin"(reference=w368) -> ("Accessors:Module ID"=w367:i32)  [unwired: 1 in, 2 out]
      n170 = call-dynamic "Delacor_lib_QMH_Release Message Queue.vi"("error in"=w375, "Message Queue"=w366) -> ("error out"=w374:errorcluster)  [unwired: 9 in]
      n171 = call "Module Name--constant.vi"("Module ID"=w367) -> ("Module Name"=w372:string)  [unwired: 10 in]
      n172 = Format Into String(format string="An error occurred during initialization. %s is no longer running.", w372) -> (resulting string=w370:string)  [unwired: 2 in, 1 out]
      n173 = call "Error Reported.vi"("Additional Information"=w370, "Error"=w374, "Module ID"=w367) -> ()  [unwired: 8 in, 1 out]
    }
  }
  n174 = Merge Errors(w17, w16) -> (w18:errorcluster)
  n175 = call "Close Module.vi"("error in"=w18, "Wait for stop?"=w2, "Module Admin in"=w4) -> ("error out"=w14:errorcluster, "External Launch"=w1:bool, "Module Admin out"=w3:refnum<class "Delacor_lib_QMH_Cloneable Module Admin.lvclass">)  [unwired: 6 in]
  n176 = Unregister For Events(event registration refnum=w9, error in=w14) -> (error out=w13:errorcluster)
  "error out" <- w13
  n177 = case "External Launch?" shown="True" w1 {
    tunnel: w13 -> [_ w376]
    frame False {
    }
    frame True {
      n178 = case shown="No Error" w376 {
        frame No Error {
          n179 = invoke class="VI" method="FP.Close"() -> ()  [unwired: 3 in, 3 out]
        }
        frame Error {
          n180 = disable-structure shown="Default" {
            frame condition #0 (active) {
              n181 = invoke class="VI" method="FP.Open"("Activate"=TRUE ("Activate?")) -> ()  [unwired: 4 in, 5 out]
            }
            frame condition #1 {
              # "Don't show panel on error if running inside a built EXE."
            }
          }
        }
      }
    }
  }
  n182 = local write "Module Admin"(w3) -> ()
